vi "test_RPLiDAR_Main5.vi"() -> ()   [LabVIEW 2019]
uses:
  Ctrl/system_hw.ctl
  Ctrl/rplidar_cmd.ctl
panel:
  out "XY 그래프 2":cluster{"X":dbl, "Y":dbl}[](graph)
  out "r-theta":cluster{"angle":dbl, "distance":dbl}[](array[cluster])
  out "n queue":i32
  out "XY 그래프":cluster{"X":dbl, "Y":dbl}[](graph)
  in  "stop":bool
  in  "RPLidar cfg":T1={"port"="COM6", "dt"=4, "update n"=44, "speed"=444, "rate "=256000} {"speed" scale=100.0..1000.0}
  in  "HW info":T2={"AGV"=enum."none", "Lidar 1"=enum."RPLidar A3", "Lidar 2"=enum."none", "GPS"=enum."none", "Camera"=enum."none", "Joystick"=enum."none", "sound"=enum."none", "IMU"=enum."none", "Led"=enum."none"}
  out "dt":u32
  out "buff chart":u32(graph)
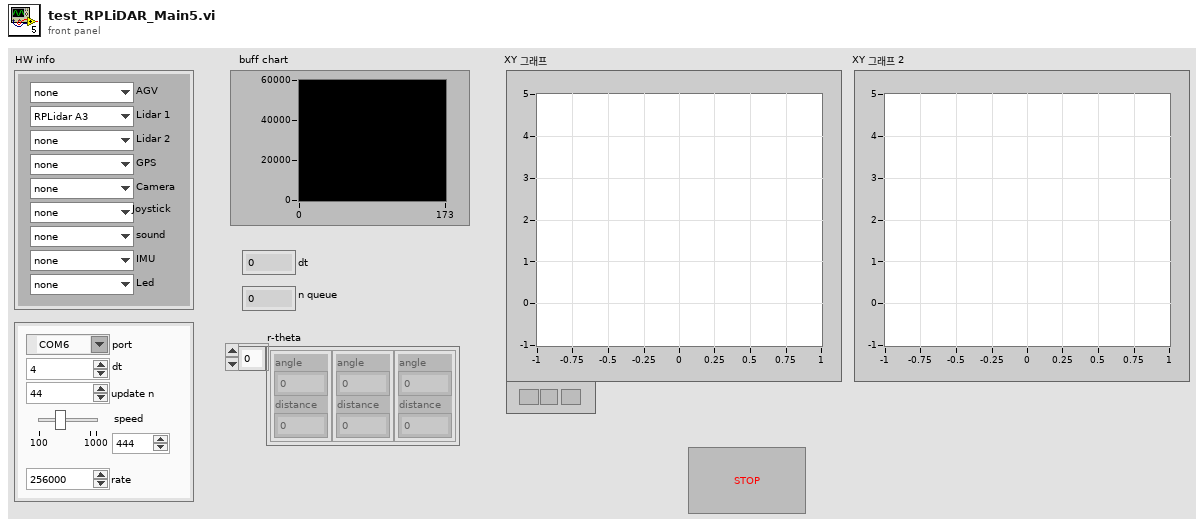
[diagram p1: front panel]
types:
  T1 = cluster{"port":refnum<visa-resource-name>, "dt":u32, "update n":u8, "speed":u16, "rate ":u32}
  T2 = typedef "system_hw.ctl" = cluster{"AGV":enum16{"none", "ERP42", "Scout", "Ycar"}, "Lidar 1":enum16{"none", "VLP16", "TIM571", "RPLidar A2", "RPLidar A3"}, "Lidar 2":enum16{"none", "VLP16", "TIM571", "RPLidar A2", "RPLidar A3"}, "GPS":enum16{"none", "F9P", "M8P", "PwrPak7", "19X HVS"}, "Camera":enum16{"none", "C920", "C922", "GT1290C", "MS LifeCam"}, "Joystick":enum16{"none", "joystick"}, "sound":enum16{"none", "speaker"}, "IMU":enum16{"none", "MW-AHRSv1"}, "Led":enum16{"none", "LedMatrix 8x32"}}
  T3 = typedef "rplidar_cmd.ctl" = enum16{"init", "health", "spin", "scan", "read", "stop", "close"}
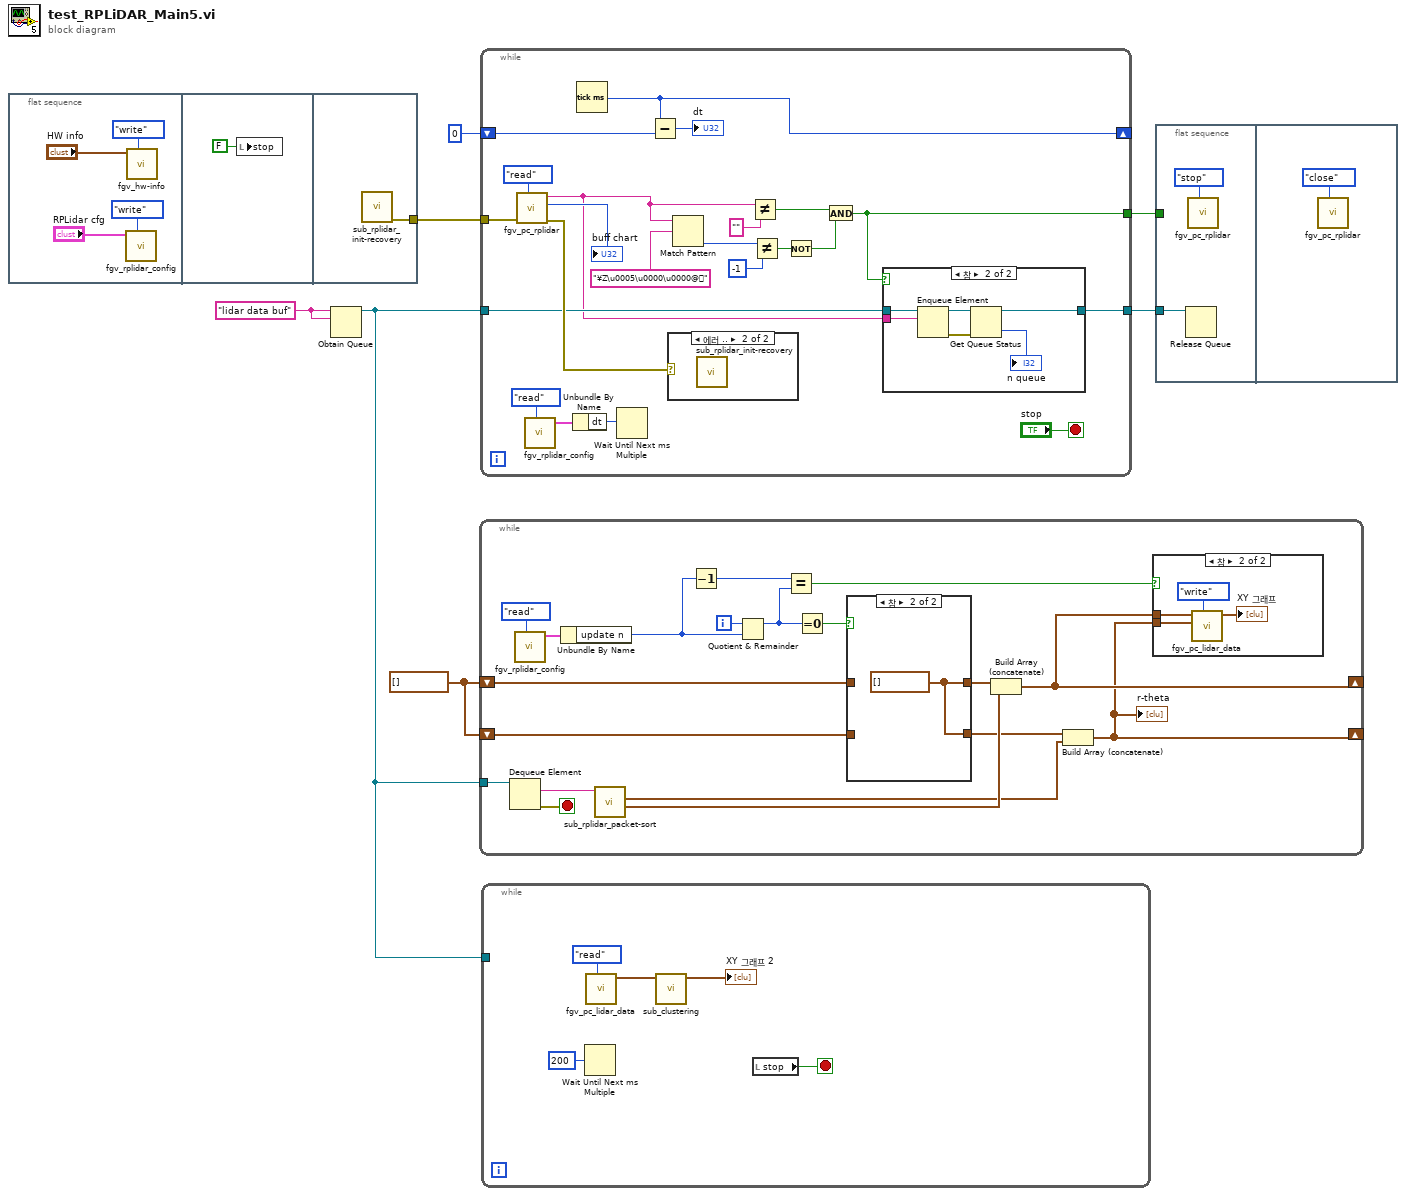
[diagram p0: block diagram]
diagram:
  w4 = "lidar data buf" ("name (unnamed)")
  w1 = cluster{dbl, dbl}[] []
  n1 = flat-sequence {
    tunnel: [w13] -> w7
    frame #0 {
      n2 = call "fgv_rplidar_config.vi"("cmd"=enum16{"read", "write"}."write", "RPLidar cfg"="RPLidar cfg") -> ()  [unwired: 8 in, 2 out]
      n3 = call "fgv_hw-info.vi"("cmd"=enum16{"write", "read"}."write", "HW info"="HW info") -> ()  [unwired: 9 in, 1 out]
    }
    frame #1 {
      n4 = local write "stop"(FALSE ("stop")) -> ()
    }
    frame #2 {
      n5 = call "sub_rplidar_init-recovery.vi"() -> ("error out"=w13:errorcluster)  [unwired: 11 in]
    }
  }
  n6 = Obtain Queue(name (unnamed)=w4, element data type=w4) -> (queue out=w2:refnum<queue>)  [unwired: 3 in, 2 out]
  n7 = while {
    shift-right: [w15] -> _
    shift-left: w1 -> [w29]
    tunnel: w2 -> [w32]
    shift-right: [w14] -> _
    shift-left: w1 -> [w17]
    i -> [w28]
    stop <- w21 stop-if-true
    n8 = Dequeue Element(queue=w32) -> (element=w31:string, error out=w21:errorcluster)  [unwired: 2 in, 2 out]
    n9 = call "fgv_rplidar_config.vi"("cmd"=enum16{"read", "write"}."read") -> ("RPLidar cfg out"=w24:T1)  [unwired: 9 in, 1 out]
    n10 = Unbundle By Name(w24) -> ("update n"=w23:u8)
    n11 = call "sub_rplidar_packet-sort.vi"("rplidar data str"=w31) -> ("xydata"=w26:cluster{"x":dbl, "y":dbl}[], "angle-distance"=w16:cluster{"angle":dbl, "distance":dbl}[])  [unwired: 8 in, 1 out]
    n12 = Decrement(x=w23) -> (x-1=w19:u8)
    n13 = Quotient & Remainder(x=w28, y=w23) -> (x-y*floor(x/y)=w20:i32)  [unwired: 1 out]
    n14 = Equal?(x=w19, y=w20) -> (x = y?=w22:bool)
    n15 = Equal To 0?(x=w20) -> (x = 0?=w27:bool)
    n16 = case shown="참" w27 {
      tunnel: [w38 w39] -> w30
      tunnel: w29 -> [w38 _]
      tunnel: [w37 w39] -> w18
      tunnel: w17 -> [w37 _]
      frame False {
      }
      frame True {
        w39 = cluster{dbl, dbl}[] []
      }
    }
    n17 = Build Array (concatenate)(w30, w26) -> (w15:cluster{"x":dbl, "y":dbl}[])
    n18 = Build Array (concatenate)(w18, w16) -> (w14:cluster{"angle":dbl, "distance":dbl}[])
    "r-theta" <- w14
    n19 = case shown="참" w22 {
      tunnel: w15 -> [_ w35]
      tunnel: w14 -> [_ w33]
      frame False {
      }
      frame True {
        n20 = call "fgv_pc_lidar_data.vi"("cmd"=enum16{"init", "read", "write"}."write", "rtheta array"=w33, "xy array"=w35) -> ("xy array out"=→"XY 그래프":cluster{"x":dbl, "y":dbl}[])  [unwired: 7 in, 1 out]
      }
    }
  }
  n21 = while {
    tunnel: w7 -> [w60]
    shift-right: [w47] -> _
    shift-left: u32 0 ("millisecond timer value") -> [w48]
    tunnel: [w42] -> w5
    tunnel: w2 -> [w43]
    tunnel: [w40] -> w3
    stop <- "stop" stop-if-true
    n22 = call "fgv_pc_rplidar.vi"("cmd"=rplidar_cmd."read", "error in"=w60) -> ("error out"=w49:errorcluster, "serial buf"=→"buff chart":u32, "read buffer"=w41:string)  [unwired: 7 in]
    n23 = call "fgv_rplidar_config.vi"("cmd"=enum16{"read", "write"}."read") -> ("RPLidar cfg out"=w51:T1)  [unwired: 9 in, 1 out]
    n24 = Unbundle By Name(w51) -> ("dt"=w50:u32)
    n25 = Tick Count (ms)() -> (millisecond timer value=w47:u32)
    n26 = Wait Until Next ms Multiple(millisecond multiple=w50) -> ()  [unwired: 1 out]
    n27 = Subtract(x=w47, y=w48) -> (x-y=→"dt":u32)
    n28 = case shown="에러 .." w49 {
      frame No Error {
      }
      frame Error {
        n29 = call "sub_rplidar_init-recovery.vi"() -> ()  [unwired: 11 in, 1 out]
      }
    }
    n30 = Match Pattern(string=w41, regular expression="¥Z\u0005\u0000\u0000@") -> (offset past match=w59:i32)  [unwired: 1 in, 3 out]
    n31 = Not Equal?(x=w41, y="") -> (x != y?=w53:bool)
    n32 = Not Equal?(x=w59, y=-1) -> (x != y?=w56:bool)
    n33 = Not(x=w56) -> (.not. x?=w54:bool)
    n34 = And(x=w53, y=w54) -> (x .and. y?=w42:bool)
    n35 = case shown="참" w42 {
      tunnel: w43 -> [w62 w68]
      tunnel: [w62 w65] -> w40
      tunnel: w41 -> [_ w66]
      frame False {
      }
      frame True {
        n36 = Enqueue Element(queue=w68, element=w66) -> (queue out=w67:refnum<queue>, error out=w64:errorcluster)  [unwired: 2 in, 1 out]
        n37 = Get Queue Status(queue=w67, error in (no error)=w64) -> (queue out=w65:refnum<queue>, # elements in queue=→"n queue":i32)  [unwired: 1 in, 6 out]
      }
    }
  }
  n38 = while {
    tunnel: w2 -> [_]
    stop <- w73 stop-if-true
    n39 = Wait Until Next ms Multiple(millisecond multiple=u32 200) -> ()  [unwired: 1 out]
    n40 = call "fgv_pc_lidar_data.vi"("cmd"=enum16{"init", "read", "write"}."read") -> ("xy array out"=w70:cluster{"x":dbl, "y":dbl}[])  [unwired: 9 in, 1 out]
    n41 = call "sub_clustering.vi"("2d data"=w70) -> ("clustering"=→"XY 그래프 2":cluster{"X":dbl, "Y":dbl}[])  [unwired: 10 in]
    n42 = local read "stop"() -> (w73:bool)
  }
  n43 = flat-sequence {
    tunnel: w5 -> [_]
    tunnel: w3 -> [w74]
    frame #0 {
      n44 = Release Queue(queue=w74) -> ()  [unwired: 2 in, 3 out]
      n45 = call "fgv_pc_rplidar.vi"("cmd"=rplidar_cmd."stop") -> ()  [unwired: 8 in, 3 out]
    }
    frame #1 {
      n46 = call "fgv_pc_rplidar.vi"("cmd"=rplidar_cmd."close") -> ()  [unwired: 8 in, 3 out]
    }
  }
